vi "mk_phi.vi"(2 "error in (no error)":errorcluster, 3 "u(t)":dbl, 4 "x(t)":dbl) -> (0 "error out":errorcluster, 1 "\\phi(t)":T1)   [LabVIEW 2021]
uses:
  <vilib>/Analysis/Matrix/Datatypes/RealMatrix.ctl
  <vilib>/Analysis/Matrix/NI_Matrix.lvlib
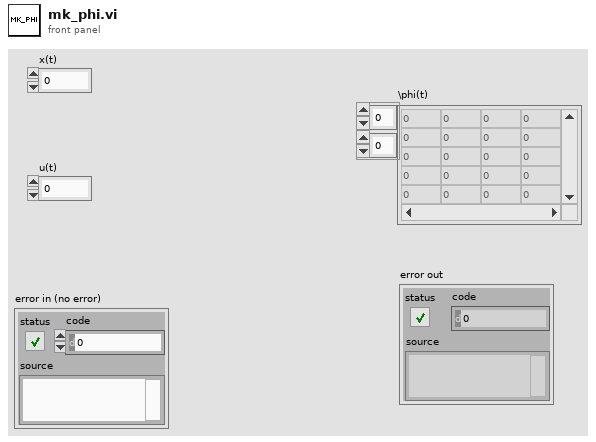
[diagram p1: front panel]
types:
  T1 = typedef "NI_Matrix.lvlib/RealMatrix.ctl" = dbl[][]
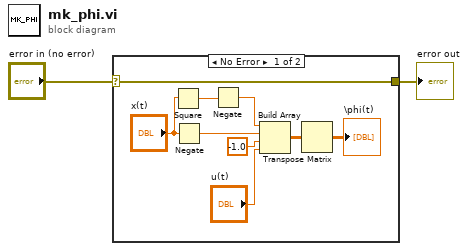
[diagram p0: block diagram]
diagram:
  n1 = case shown="No Error" "error in (no error)" {
    selector: "error in (no error)" -> [w5 w12]
    tunnel: [w5 w12] -> w1
    frame No Error {
      n2 = Square(x="x(t)") -> (x^2=w10:dbl)
      n3 = Negate(x="x(t)") -> (-x=w8:dbl)
      n4 = Negate(x=w10) -> (-x=w11:dbl)
      n5 = Build Array(w11, w8, -1.0, "u(t)") -> (w4:T1)
      n6 = Transpose Matrix(1:w4) -> (0:→"\\phi(t)":T1)
    }
    frame Error {
    }
  }
  "error out" <- w1
